vi "Forward Move 2.vi"   [LabVIEW 2012]
uses:
  <vilib>/Instr/_visa.llb/VISA Configure Serial Port (Instr).vi
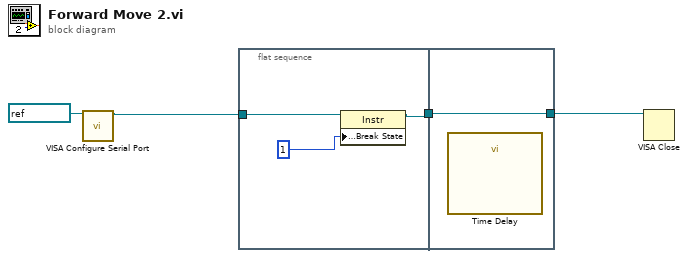
[diagram p0: block diagram]
diagram:
  n1 = call-poly "VISA Configure Serial Port"("VISA resource name"=refnum<visa-resource-name> "COM1") -> ("VISA resource name out"=w3:refnum<visa-resource-name>)  [unwired: 5 in, 9 out]
  n2 = flat-sequence {
    tunnel: w3 -> [w6]
    tunnel: [w5] -> w1
    tunnel: [w8] -> w2
    tunnel: w1 -> [w8]
    frame #0 {
      n3 = property class="Instr"(reference=w6, "Serial Settings:Modem Line Settings:Break State"=1) -> (reference out=w5:refnum<visa-resource-name>)  [unwired: 1 in, 1 out]
    }
    frame #1 {
      n4 = call "Time Delay"() -> ()  [unwired: 2 in, 10 out]
    }
  }
  n5 = VISA Close(VISA resource name=w2) -> ()  [unwired: 1 in, 1 out]
